vi "Gen_Stat_Array.vi"(8 "error in (no error)":errorcluster, 10 "Array":string[](array[string]), 11 "User Event in":refnum<user-event>) -> (0 "error out":errorcluster, 3 "User Event out":refnum<user-event>)   [LabVIEW 2014, in "UserEvent.lvlib"]
uses:
  Main/TypeDef/EventData.ctl
  UserEvent.lvlib
  Main/Main.lvlib
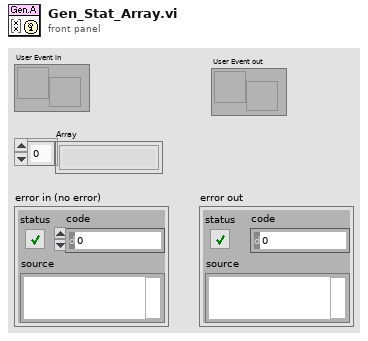
[diagram p1: front panel]
types:
  T1 = typedef "Main.lvlib/EventData.ctl" = cluster{"State":string, "Data":variant}
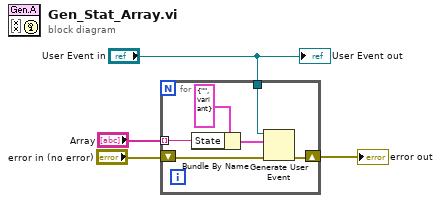
[diagram p0: block diagram]
diagram:
  n1 = for {
    tunnel: "User Event in" -> [w7]
    shift-right: [w6] -> w4
    shift-left: "error in (no error)" -> [w8]
    tunnel: "Array" -> [w5] mode=indexing
    n2 = Bundle By Name(cluster=T1 {"State"="", "Data"=variant} ("event data"), "State"=w5) -> (w9:T1)
    n3 = Generate User Event(user event=w7, event data cluster=w9, error in=w8) -> (error out=w6:errorcluster)  [unwired: 1 in, 1 out]
  }
  "error out" <- w4
  "User Event out" <- "User Event in"
